vi "Graph Properties Runtime.vi"(0 "Long Term Graph":refnum<vi>, 7 "Selected Variables":string[][](array[string]), 9 "Plot Data":dbl[](array[numeric]), 11 "error in (no error)":errorcluster) -> (15 "error out":errorcluster)   [LabVIEW 2020]
doc: "This vi change the graph properties during runtime and displays runtime plot data in plot names\n[Input]\nLong term plot reference\nSelected variables array\nPlot data\nError in\n[output]\nerror out"
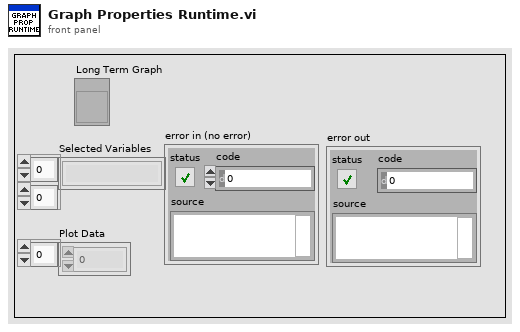
[diagram p1: front panel]
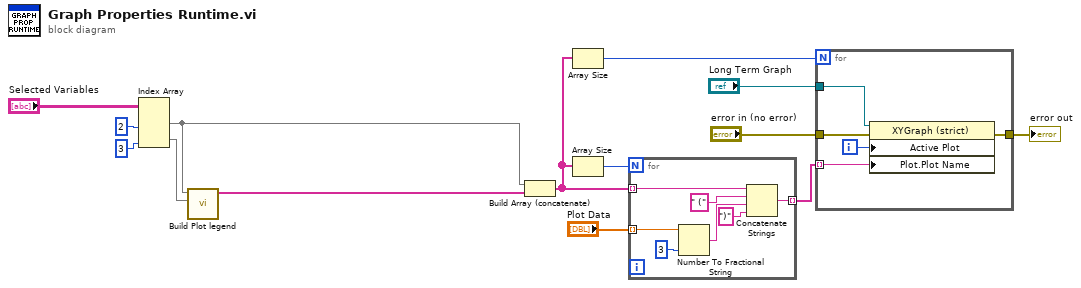
[diagram p0: block diagram]
diagram:
  n1 = Index Array(array="Selected Variables", index (col) #1=2 ("disabled index (col)"), index (col) #2=3 ("index (col)")) -> (element #1=w1:string[], element #2=w3:string[])  [unwired: 2 in]
  n2 = call "Build Plot legend.vi"("Reference Values"=w3, "Display Names"=w1) -> ("Plot legend Names"=w2:string[])  [unwired: 8 in, 1 out]
  n3 = Build Array (concatenate)(w1, w2) -> (w6:string[])
  n4 = Array Size(array=w6) -> (size(s)=w7:i32)
  n5 = Array Size(array=w6) -> (size(s)=w13:i32)
  n6 = for {
    N: w13 -> [_]
    tunnel: "Plot Data" -> [w21] mode=indexing
    tunnel: w6 -> [w15] mode=indexing
    tunnel: [w20] -> w12 mode=indexing
    n7 = Number To Fractional String(number=w21, precision (6)=i16 3) -> (F-format string=w17:string)  [unwired: 2 in]
    n8 = Concatenate Strings(w15, " (" ("string"), w17, ")" ("string")) -> (w20:string)
  }
  n9 = for {
    N: w7 -> [_]
    tunnel: "Long Term Graph" -> [w26]
    tunnel: w12 -> [w25] mode=indexing
    tunnel: "error in (no error)" -> [w24]
    tunnel: [w23] -> w5
    i -> [w22]
    n10 = property class="XYGraph (strict)"(reference=w26, error in=w24, "Active Plot"=w22, "Plot.Plot Name"=w25) -> (error out=w23:errorcluster)  [unwired: 1 out]
  }
  "error out" <- w5
